vi "formate indice revision client.vi"(0 "Indice révision client IN":string) -> (1 "Indice révision client text":string, 2 "Indice révision client OUT":string)   [LabVIEW 2020]
doc: "Prend l'indice client de la base de données.\nS'il n'y en a pas, renvoie \"00\"."
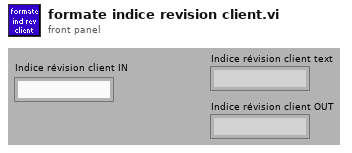
[diagram p1: front panel]
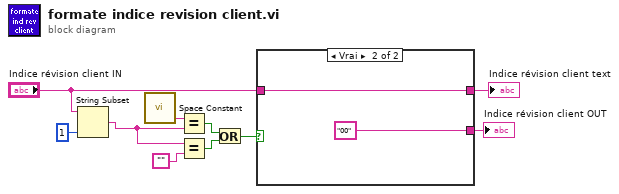
[diagram p0: block diagram]
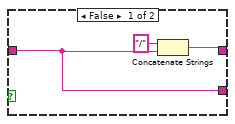
[diagram p2: hidden frame]
diagram:
  n1 = String Subset(string="Indice révision client IN", length (rest)=1 ("longueur (reste)")) -> (substring=w2:string)  [unwired: 1 in]
  n2 = call <vilib>:"Space Constant.vi"() -> ("String"=w9:string)
  n3 = Equal?(x=w9, y=w2) -> (x = y?=w7:bool)
  n4 = Equal?(x=w2, y="") -> (x = y?=w8:bool)
  n5 = Or(x=w7, y=w8) -> (x .or. y?=w6:bool)
  n6 = case shown="Vrai" w6 {
    tunnel: "Indice révision client IN" -> [w12 w14]
    tunnel: [w12 "00"] -> w5
    tunnel: [w11 w14] -> w1
    frame False {
      n7 = Concatenate Strings("/" ("chaîne"), w12) -> (w11:string)
    }
    frame True {
    }
  }
  "Indice révision client OUT" <- w5
  "Indice révision client text" <- w1
